vi "Eurotherm - VISA Serial - Initialize Session.vi"(0 "Communication":T1={"Com Port"=1, "Address"=1, "Baud Rate"=9600} {"Baud Rate" items=["300"=300, "600"=600, "1200"=1200, "2400"=2400, "4800"=4800, "9600 (default)"=9600, "19200"=19200, "38400"=38400, "57600"=57600, "76800"=76800, "115200"=115200, "230400"=230400]; "Com Port" min=1 max=255; "Address" min=1 max=99}, 11 "error in (no error)":errorcluster) -> (4 "VISA":refnum<visa-resource-name>, 15 "error out":errorcluster)   [LabVIEW 2011]
uses:
  Eurotherm - Controls/Eurotherm - Communication.ctl
  Common/Utilities/Controls - Com Ports/Com Port - Numeric.ctl
  Eurotherm - Controls/Eurotherm - Address.ctl
  Common/Utilities/Controls - Com Ports/Com Port - Baud Rate.ctl
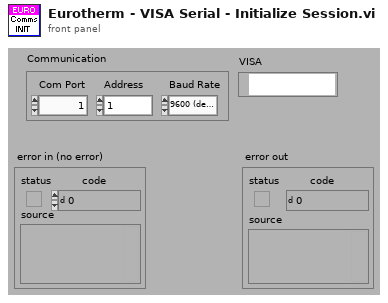
[diagram p1: front panel]
types:
  T1 = typedef "Eurotherm - Communication.ctl" = cluster{"Com Port":T2, "Address":T3, "Baud Rate":T4}
  T2 = typedef "Com Port - Numeric.ctl" = i32
  T3 = typedef "Eurotherm - Address.ctl" = u8
  T4 = typedef "Com Port - Baud Rate.ctl" = u32
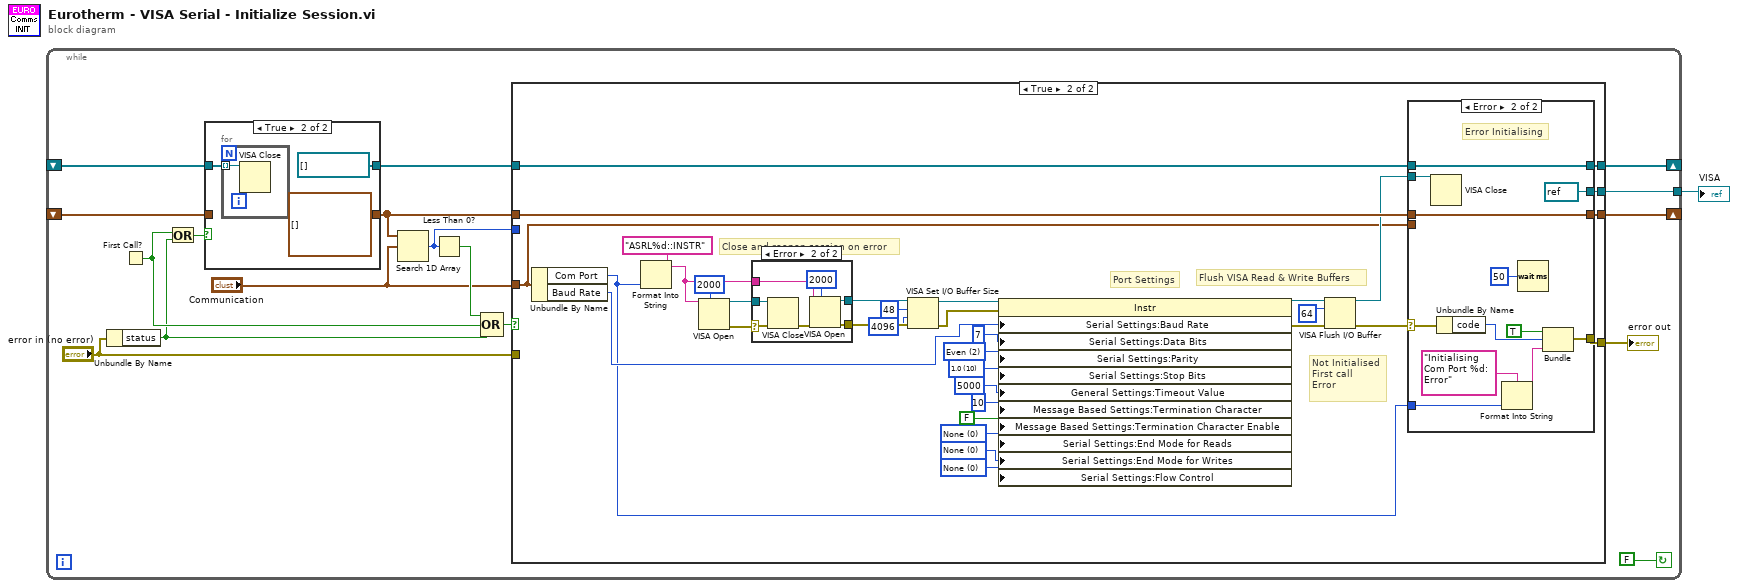
[diagram p0: block diagram]
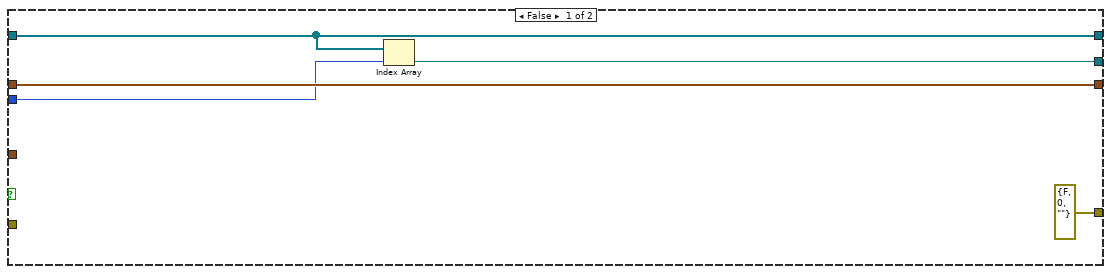
[diagram p3: hidden frame]
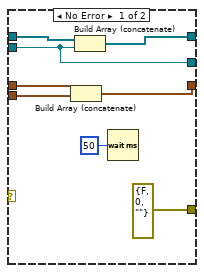
[diagram p5: hidden frame]
diagram:
  n1 = while {
    shift-right: [w18] -> _
    shift-left: _ -> [w17]
    shift-right: [w4] -> _
    shift-left: _ -> [w6]
    tunnel: [w2] -> w1
    stop <- FALSE continue-if-true
    n2 = Unbundle By Name("error in (no error)") -> ("status"=w11:bool)
    n3 = First Call?() -> (First Call?: T/F=w12:bool)
    n4 = Or(x=w12, y=w11) -> (x .or. y?=w10:bool)
    n5 = case shown="True" w10 {
      tunnel: [w20 T1[] []] -> w15
      tunnel: w17 -> [w20 _]
      tunnel: w6 -> [w19 w21]
      tunnel: [w19 refnum<visa-resource-name>[] []] -> w5
      frame False {
      }
      frame True {
        n6 = for {
          tunnel: w21 -> [w24] mode=indexing
          n7 = VISA Close(VISA resource name=w24) -> ()  [unwired: 1 in, 1 out]
        }
      }
    }
    n8 = Search 1D Array(1D array=w15, element="Communication") -> (index of element=w3:i32)  [unwired: 1 in]
    n9 = Less Than 0?(x=w3) -> (x < 0?=w13:bool)
    n10 = Compound Arithmetic op=OR(w13, w12, w11) -> (w14:bool)
    n11 = case shown="True" w14 {
      tunnel: [w29 w63] -> w18
      tunnel: w15 -> [w29 w62]
      tunnel: "Communication" -> [_ w31]
      tunnel: [cluster{bool, "error code":i32, string} {FALSE, "error code"=0, ""} w61] -> w9
      tunnel: "error in (no error)" -> [_ _]
      tunnel: w5 -> [w27 w46]
      tunnel: [w27 w45] -> w4
      tunnel: w3 -> [w26 _]
      tunnel: [w25 w42] -> w2
      frame False {
        n12 = Index Array(array=w27, index=w26) -> (element=w25:refnum<visa-resource-name>)
      }
      frame True {
        w59 = u16 0 items=["None", "XON/XOFF", "RTS/CTS", "XON/XOFF & RTS/CTS", "DTR/DSR", "XON/XOFF & DTR/DSR"] ("Serial Settings:Serial Flow Control")
        w58 = u16 0 items=["None", "LastBit", "TermChar", "Break"] ("Serial Settings:Serial End Mode for Writes")
        w57 = u16 0 items=["None", "LastBit", "TermChar"] ("Serial Settings:Serial End Mode for Reads")
        w56 = u16 2 items=["None", "Odd", "Even", "Mark", "Space"] ("Serial Settings:Serial Parity")
        w54 = u16 10 items=["1.0"=10, "1.5"=15, "2.0"=20] ("Serial Settings:Serial Stop Bits")
        # "Close and reopen session on error"
        # "Port Settings"
        # "Flush VISA Read & Write Buffers"
        # "Not Initialised\nFirst call\nError"
        n13 = Unbundle By Name(w31) -> ("Com Port"=w30:T2, "Baud Rate"=w32:T4)
        n14 = Format Into String(format string="ASRL%d::INSTR", w30) -> (resulting string=w40:string)  [unwired: 2 in, 1 out]
        n15 = VISA Open(timeout (0)=u32 2000 ("VISA Open timeout (0)"), VISA resource name=w40) -> (VISA resource name=w48:refnum<visa-resource-name>, error out=w47:errorcluster)  [unwired: 3 in]
        n16 = case shown="Error" w47 {
          selector: w47 -> [w64 w68]
          tunnel: w48 -> [w65 w72]
          tunnel: [w65 w70] -> w38
          tunnel: [w64 w69] -> w37
          tunnel: w40 -> [_ w67]
          frame No Error {
          }
          frame Error {
            n17 = VISA Close(VISA resource name=w72, error in (no error)=w68) -> (error out=w71:errorcluster)
            n18 = VISA Open(timeout (0)=u32 2000 ("VISA Open timeout (0)"), error in (no error)=w71, VISA resource name=w67) -> (VISA resource name=w70:refnum<visa-resource-name>, error out=w69:errorcluster)  [unwired: 2 in]
          }
        }
        n19 = VISA Set I/O Buffer Size(VISA resource name=w38, mask (16)=u16 48, size (4096)=u32 4096, error in (no error)=w37) -> (VISA resource name out=w35:refnum<visa-resource-name>, error out=w36:errorcluster)
        n20 = property class="Instr"(reference=w35, error in=w36, "Serial Settings:Baud Rate"=w32, "Serial Settings:Data Bits"=u16 7 ("Serial Settings:Serial Data Bits"), "Serial Settings:Parity"=w56, "Serial Settings:Stop Bits"=w54, "General Settings:Timeout Value"=u32 5000 ("Timeout"), "Message Based Settings:Termination Character"=u8 10 ("Termination Character"), "Message Based Settings:Termination Character Enable"=FALSE ("Termination Character Enable"), "Serial Settings:End Mode for Reads"=w57, "Serial Settings:End Mode for Writes"=w58, "Serial Settings:Flow Control"=w59) -> (reference out=w49:refnum<visa-resource-name>, error out=w50:errorcluster)
        n21 = VISA Flush I/O Buffer(VISA resource name=w49, mask (16)=u16 64, error in (no error)=w50) -> (VISA resource name out=w43:refnum<visa-resource-name>, error out=w44:errorcluster)
        n22 = case shown="Error" w44 {
          selector: w44 -> [_ w81]
          tunnel: [w77 w83] -> w63
          tunnel: w31 -> [w78 _]
          tunnel: w62 -> [w79 w83]
          tunnel: [cluster{bool, "error code":i32, string} {FALSE, "error code"=0, ""} w92] -> w61
          tunnel: w30 -> [_ w89]
          tunnel: w43 -> [w74 w85]
          tunnel: w46 -> [w76 w84]
          tunnel: [w75 w84] -> w45
          tunnel: [w74 refnum<visa-resource-name> refnum ("Com Port Number")] -> w42
          frame No Error {
            n23 = Build Array (concatenate)(w79, w78) -> (w77:T1[])
            n24 = Build Array (concatenate)(w76, w74) -> (w75:refnum<visa-resource-name>[])
            n25 = Wait (ms)(milliseconds to wait=u32 50) -> ()  [unwired: 1 out]
          }
          frame Error {
            # "Error Initialising"
            n26 = VISA Close(VISA resource name=w85) -> ()  [unwired: 1 in, 1 out]
            n27 = Unbundle By Name(w81) -> ("code"=w87:i32)
            n28 = Format Into String(format string="Initialising Com Port %d: Error", w89) -> (resulting string=w88:string)  [unwired: 2 in, 1 out]
            n29 = Wait (ms)(milliseconds to wait=u32 50) -> ()  [unwired: 1 out]
            n30 = Bundle(TRUE, "code"=w87, w88) -> (w92:cluster{bool, "code":i32, string})  [unwired: 1 in]
          }
        }
      }
    }
    "error out" <- w9
  }
  "VISA" <- w1
